vi "Set Bit Value.vi"(6 "BitValue":bool, 7 "BitPosition":T1(ring), 10 "Data In":u8 format="%08b") -> (2 "Data Out":u8 format="%08b")   [LabVIEW 2011]
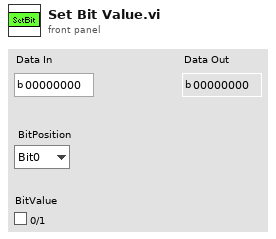
[diagram p1: front panel]
types:
  T1 = enum16{"Bit0", "Bit1", "Bit2", "Bit3", "Bit4", "Bit5", "Bit6", "Bit7"}
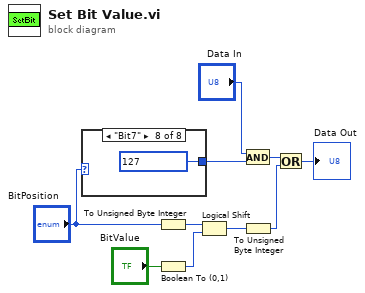
[diagram p0: block diagram]
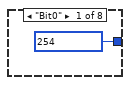
[diagram p2: hidden frame]
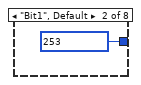
[diagram p3: hidden frame]
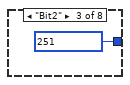
[diagram p4: hidden frame]
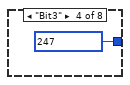
[diagram p5: hidden frame]
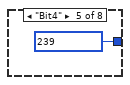
[diagram p6: hidden frame]
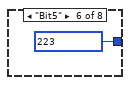
[diagram p7: hidden frame]
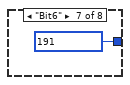
[diagram p8: hidden frame]
diagram:
  n1 = case shown="\"Bit7\"" "BitPosition" {
    tunnel: [u8 254 ("Data") u8 253 ("Data") u8 251 ("Data") u8 247 ("Data") u8 239 ("Data") u8 223 ("Data") u8 191 ("Data") u8 127 ("Data")] -> w9
    frame "Bit0" {
    }
    frame "Bit1", Default {
    }
    frame "Bit2" {
    }
    frame "Bit3" {
    }
    frame "Bit4" {
    }
    frame "Bit5" {
    }
    frame "Bit6" {
    }
    frame "Bit7" {
    }
  }
  n2 = To Unsigned Byte Integer(number="BitPosition") -> (unsigned 8bit integer=w7:u8)
  n3 = Boolean To (0,1)(Boolean="BitValue") -> (0, 1=w5:i16)
  n4 = Logical Shift(y=w7, x=w5) -> (x << y=w3:i16)
  n5 = And(x="Data In", y=w9) -> (x .and. y?=w8:u8)
  n6 = To Unsigned Byte Integer(number=w3) -> (unsigned 8bit integer=w1:u8)
  n7 = Or(x=w8, y=w1) -> (x .or. y?=→"Data Out":u8)
